vi "Main.vi"(11 "Module Admin":refnum<class "Delacor_lib_QMH_Module Admin.lvclass">) -> ()   [LabVIEW 2019, in "ContextHelp.lvlib"]
doc: "This template is based off of the Queued Message Handler design pattern and the Queued Message Handler project template that ships with LabVIEW.\n\nThe main difference is that the queue is private to this module and communication between modules is performed via Broadcast and Request events.\n\nRequest events are wrapped in public API methods and are handled in the Event Handling Loop (EHL) of this VI. Any module can register for Broadcast events sent by this module. The EHL generates messages based on user interface actions.\n\nThe Message Handling Loop (MHL) processes messages generated by the EHL, or by other messages. The messages are string values, so new messages can be added easily to the Message Cases case structure in the MHL. Each message cluster can also provide an optional value for Message Data, which is a variant that can be converted to whatever message-specific data is required.\n_____\nBased on DQMH Project Template 6.1.0.94.\n____\nPantherLAB Templates 1.0.0.5\nCopyright (c) 2022, PantherLAB"
uses:
  ContextHelp.lvlib
  <vilib>/Delacor/Delacor QMH/Libraries/Module Admin_class/Delacor_lib_QMH_Module Admin.lvclass
  Module Data--cluster.ctl
  <vilib>/Delacor/Delacor QMH/Libraries/Message Queue_class/Delacor_lib_QMH_Message Queue.lvclass/Delacor_lib_QMH_Message Queue.ctl
  Stop Argument--cluster.ctl
  <vilib>/Delacor/Delacor QMH/Libraries/Module Admin_class/Delacor_lib_QMH_Module Admin.lvclass/Delacor_lib_QMH_Module Admin.ctl
  Draw Panel Into Subpanel Argument--cluster.ctl
  Remove Panel from Subpanel Argument--cluster.ctl
  <vilib>/Delacor/Delacor QMH/Libraries/Message Queue_class/Delacor_lib_QMH_Enqueue Message (Single).vi
  <vilib>/Delacor/Delacor QMH/Libraries/Module Admin_class/Delacor_lib_QMH_Get External Launch.vi
  <vilib>/Utility/error.llb/Error Cluster From Error Code.vi
  <vilib>/ErrorRing/Error Ring.xnode
  <vilib>/Delacor/Delacor QMH/Libraries/Message Queue_class/Delacor_lib_QMH_Message Queue.lvclass
  Panther Dashboard/Panther Dashboard.lvlib
panel:
  out "Status":string
  out "error out":errorcluster
  out "DQMH Version":string
  in  "Edit Project Description":bool caption="Project Description"
  in  "Project Description":string
  in  "Edit Module Description":bool caption="Module Description"
  in  "Module Description":string
  in  "Edit VI":bool caption="Event Description"
  out "Event Connector Pane":picture
  in  "Event Description":string
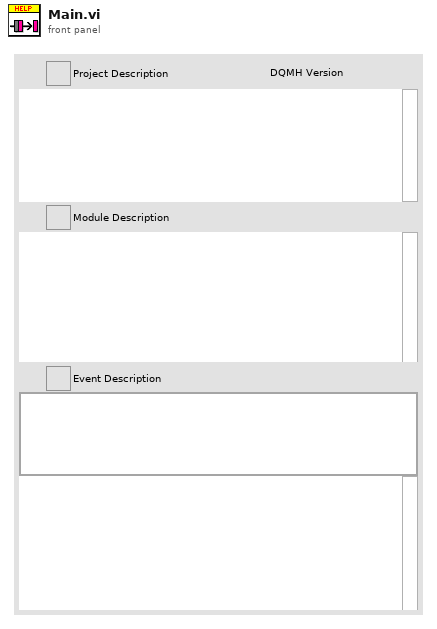
[diagram p1: front panel]
types:
  T1 = typedef "Panther Dashboard.lvlib/Broadcast Events--cluster.ctl" = cluster{"Module Did Init":refnum<user-event>, "Status Updated":refnum<user-event>, "Error Reported":refnum<user-event>, "Module Did Stop":refnum<user-event>, "Update Module Execution Status":refnum<user-event>, "References Updated":refnum<user-event>, "Projects Updated":refnum<user-event>, "Targets Updated":refnum<user-event>, "Progress updated":refnum<user-event>, "Scale Updated":refnum<user-event>, "Connector Pane Updated":refnum<user-event>, "Documentation Updated":refnum<user-event>, "Module Type Updated":refnum<user-event>, "Theme Updated":refnum<user-event>, "Project Description Updated":refnum<user-event>}
  T2 = typedef "ContextHelp.lvlib/Request Events--cluster.ctl" = cluster{"Stop Module":refnum<user-event>, "Show Panel":refnum<user-event>, "Hide Panel":refnum<user-event>, "Get Module Execution Status":refnum<user-event>, "Show Diagram":refnum<user-event>, "Draw Panel Into Subpanel":refnum<user-event>, "Remove Panel from Subpanel":refnum<user-event>, "Refresh Panther Dashboard Broadcasts":refnum<user-event>}
  T3 = typedef "ContextHelp.lvlib/Module Data--cluster.ctl" = cluster{"Status":string, "SubPanel":refnum<vi>, "Panel Status":bool}
  T4 = enum8{"Enabled", "Disabled", "Disabled and Grayed Out"}
  T5 = enum32{"invalid lock state", "Not Locked", "Locked (No Password)", "Password-protected"}
  T6 = typedef "ContextHelp.lvlib/Stop Argument--cluster.ctl" = cluster{"Origin":string, "Exit via Stop Module Req?":bool, "Wait for Module to stop?":bool}
  T7 = typedef "ContextHelp.lvlib/Draw Panel Into Subpanel Argument--cluster.ctl" = cluster{"Sub Panel":refnum<vi>}
  T8 = typedef "ContextHelp.lvlib/Remove Panel from Subpanel Argument--cluster.ctl" = cluster{"Boolean":bool}
  T9 = enum32{"Invalid", "Standard", "Closed", "Hidden", "Minimized", "Maximized"}
  T10 = typedef "Panther Dashboard.lvlib/Documentation--cluster.ctl" = cluster{"Module Description":string, "Event Description":string}
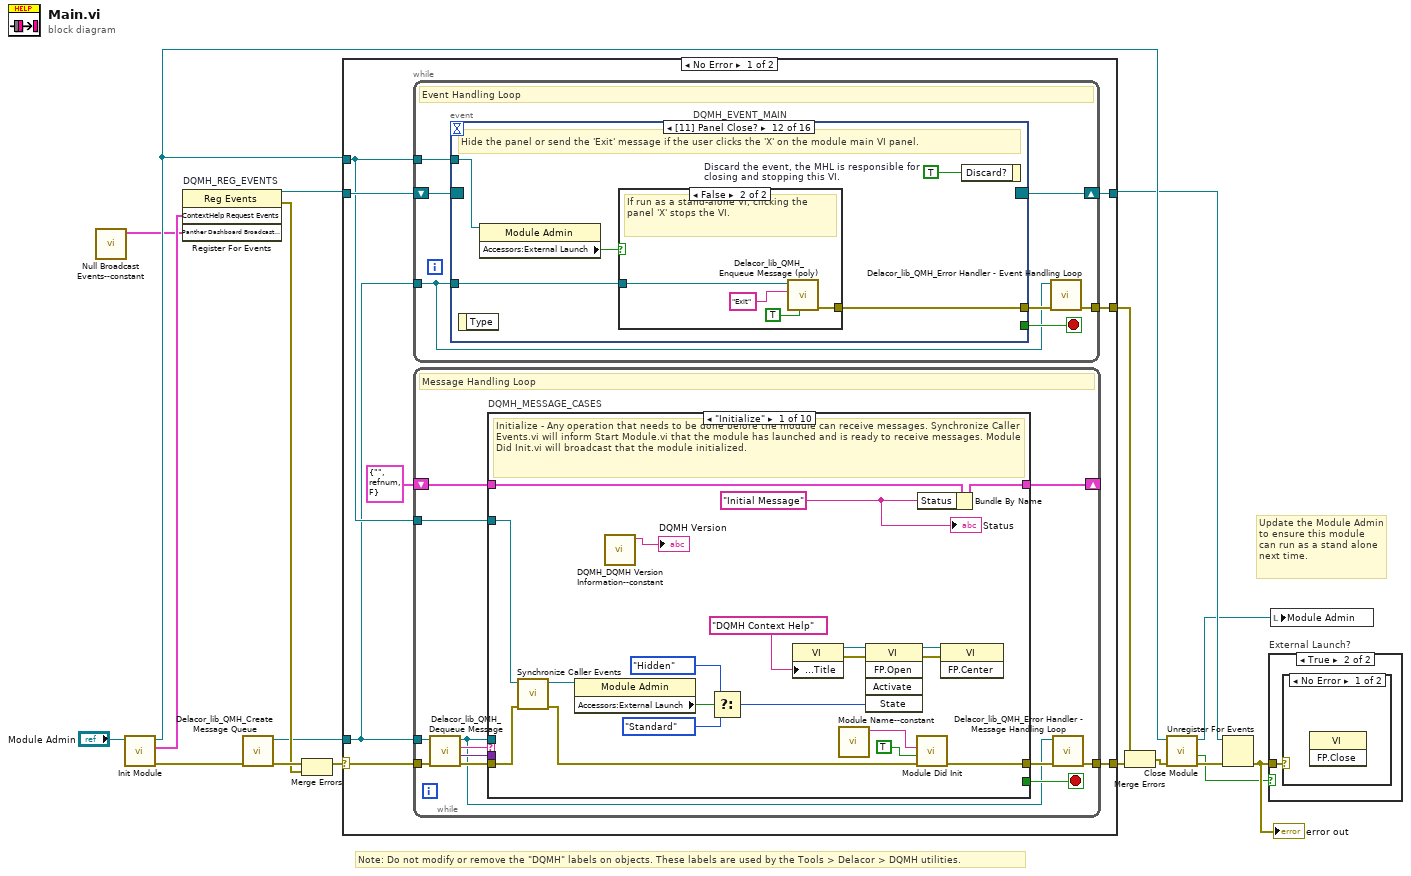
[diagram p0: block diagram]
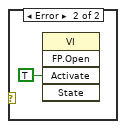
[diagram p3: hidden frame]
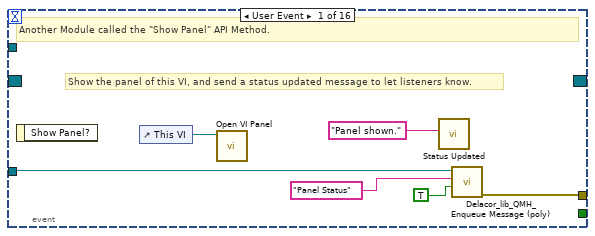
[diagram p4: hidden frame]
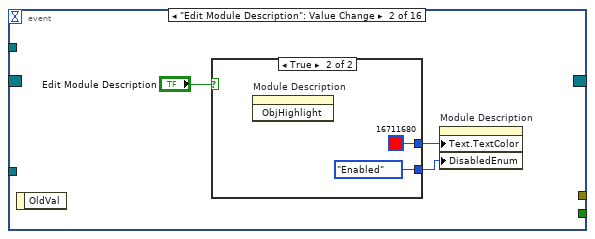
[diagram p5: hidden frame]
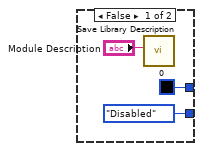
[diagram p6: hidden frame]
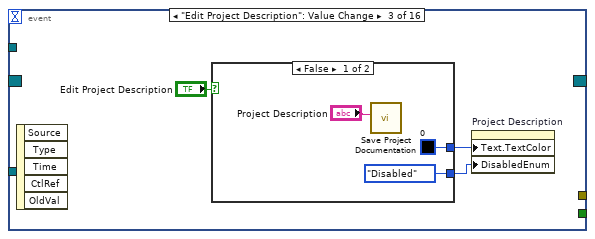
[diagram p7: hidden frame]
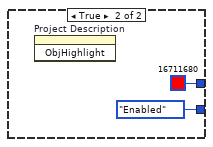
[diagram p8: hidden frame]
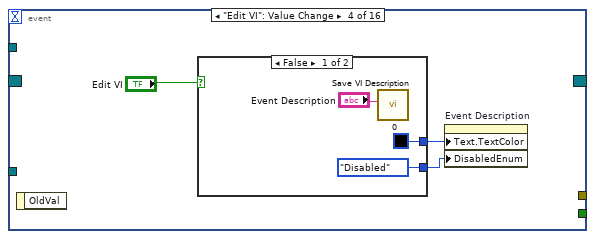
[diagram p9: hidden frame]
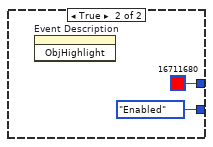
[diagram p10: hidden frame]
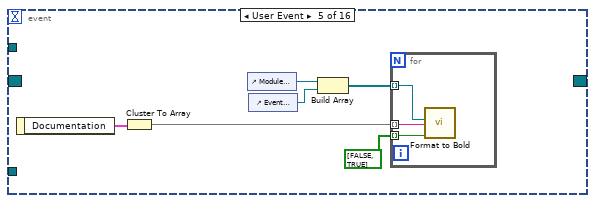
[diagram p11: hidden frame]
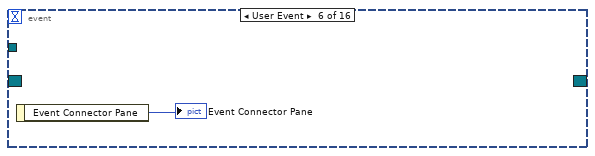
[diagram p12: hidden frame]
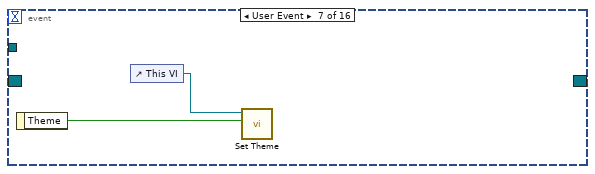
[diagram p13: hidden frame]
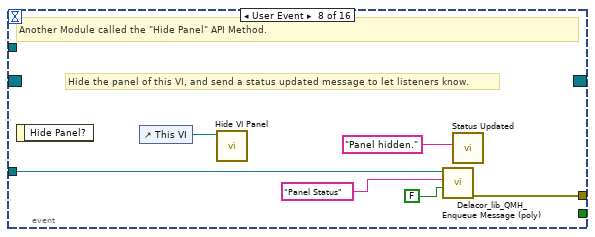
[diagram p14: hidden frame]
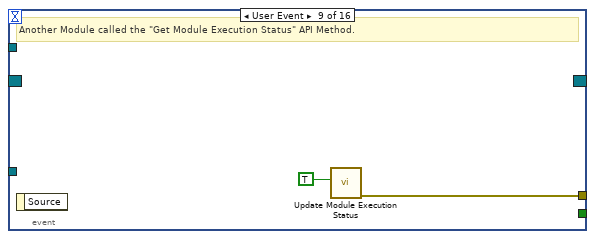
[diagram p15: hidden frame]
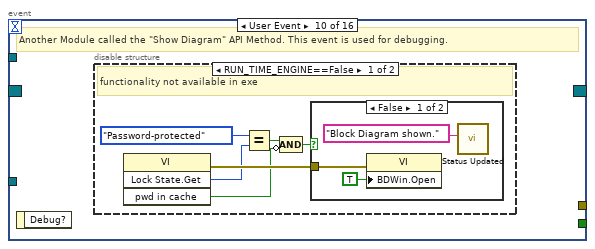
[diagram p16: hidden frame]
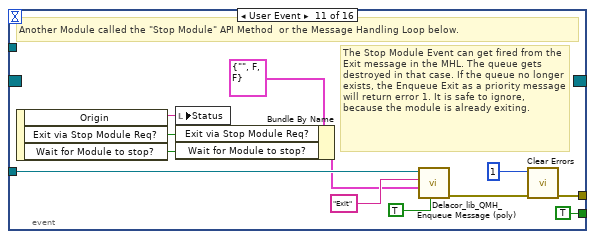
[diagram p19: hidden frame]
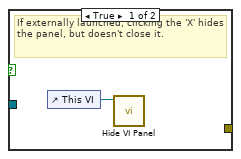
[diagram p20: hidden frame]
diagram:
  # "Note: Do not modify or remove the \"DQMH\" labels on objects. These labels are used by the Tools > Delacor > DQMH utilities."
  # "Update the Module Admin to ensure this module can run as a stand alone next time."
  n1 = call "Null Broadcast Events--constant.vi"() -> ("Panther Dashboard Broadcast Events"=w1:T1)  [unwired: 11 in]
  n2 = call "Init Module.vi"("Singleton Module Admin in"="Module Admin") -> ("error out"=w17:errorcluster, "ContextHelp Request Events"=w2:T2, "Singleton Module Admin out"=w9:refnum<class "Delacor_lib_QMH_Module Admin.lvclass">)  [unwired: 8 in]
  n3 = register-events "DQMH_REG_EVENTS"(w2, w1) -> (reference out=w7:refnum<event-registration>, error out=w10:errorcluster)  [unwired: 2 in]
  n4 = call <vilib>:"Delacor_lib_QMH_Create Message Queue.vi"("error in"=w17) -> ("error out"=w12:errorcluster, "Message Queue"=w6:refnum<class "Delacor_lib_QMH_Message Queue.lvclass">)  [unwired: 9 in]
  n5 = Merge Errors(w12, w10) -> (w11:errorcluster)
  n6 = case shown="No Error" w11 {
    selector: w11 -> [w24 w252]
    tunnel: [w26 w251] -> w18
    tunnel: [w23 w250] -> w8
    tunnel: w7 -> [w21 w250]
    tunnel: w6 -> [w19 w245]
    tunnel: [w25 _] -> w15
    tunnel: w9 -> [w20 w246]
    frame No Error {
      n7 = while {
        tunnel: w19 -> [w27]
        shift-right: [w30] -> w23
        shift-left: w21 -> [w31]
        tunnel: [w32] -> w25
        tunnel: w20 -> [w28]
        stop <- w29 stop-if-true
        # "Event Handling Loop"
        n8 = event "DQMH_EVENT_MAIN" shown="[11] Panel Close?" {
          selector: w31 -> [_ _ _ _ _ _ _ _ _ _ _ _ _ _ w129 _]
          dyn-events: [_ _ _ _ _ _ _ _ _ _ _ _ _ _ w128 _] -> w30
          timeout: _ -> [_ _ _ _ _ _ _ _ _ _ _ _ _ _ _ _]
          tunnel: [_ _ _ _ _ _ _ _ _ _ TRUE ("Discard?") _ _ _ _ _] -> w29
          tunnel: w27 -> [w36 _ _ _ _ _ _ w76 _ _ w100 w107 w119 w125 _ _]
          tunnel: [w39 _ _ _ _ _ _ w81 w83 _ w103 w109 w120 w126 _ _] -> w33
          tunnel: w28 -> [_ _ _ _ _ _ _ _ _ _ _ w106 _ _ _ _]
          event User Event {
            # "Show the panel of this VI, and send a status updated message to let listeners know."
            # "Another Module called the \"Show Panel\" API Method."
            n9 = event-data() -> ()  [unwired: 1 in, 1 out]
            n10 = control-ref of="This VI"() -> (w38:refnum<vi>)
            n11 = call "Open VI Panel.vi"("VI"=w38) -> ()  [unwired: 10 in, 1 out]
            n12 = call "Status Updated.vi"("Status"="Panel shown." ("format string")) -> ()  [unwired: 10 in, 1 out]
            n13 = call-poly <vilib>:"Delacor_lib_QMH_Enqueue Message (poly).vi"("Message Data"=TRUE, "Message"="Panel Status" ("format string"), "Message Queue in"=w36) -> ("error out"=w39:errorcluster)  [unwired: 7 in, 1 out]
          }
          event "Edit Module Description": Value Change {
            n14 = event-data() -> ()  [unwired: 1 in, 1 out]
            n15 = case shown="True" "Edit Module Description" {
              tunnel: [u32 0 u32 16711680] -> w41
              tunnel: [T4."Disabled" ("Disabled") T4."Enabled" ("Disabled")] -> w42
              frame False {
                n16 = call "Save Library Description.vi"("Library Description"="Module Description") -> ()  [unwired: 10 in, 1 out]
              }
              frame True {
                n17 = invoke on="Module Description" class="Str" method="ObjHighlight"() -> ()  [unwired: 3 in, 3 out]
              }
            }
            n18 = property on="Module Description" class="Str"("Text.TextColor"=w41, "DisabledEnum"=w42) -> ()  [unwired: 2 in, 2 out]
          }
          event "Edit Project Description": Value Change {
            n19 = event-data() -> ()  [unwired: 1 in, 5 out]
            n20 = case shown="False" "Edit Project Description" {
              tunnel: [u32 0 u32 16711680] -> w49
              tunnel: [T4."Disabled" ("Disabled") T4."Enabled" ("Disabled")] -> w50
              frame False {
                n21 = call "Save Project Documentation.vi"("Project Description"="Project Description") -> ()  [unwired: 10 in, 1 out]
              }
              frame True {
                n22 = invoke on="Project Description" class="Str" method="ObjHighlight"() -> ()  [unwired: 3 in, 3 out]
              }
            }
            n23 = property on="Project Description" class="Str"("Text.TextColor"=w49, "DisabledEnum"=w50) -> ()  [unwired: 2 in, 2 out]
          }
          event "Edit VI": Value Change {
            n24 = event-data() -> ()  [unwired: 1 in, 1 out]
            n25 = case shown="False" "Edit VI" {
              tunnel: [u32 0 u32 16711680] -> w57
              tunnel: [T4."Disabled" ("Disabled") T4."Enabled" ("Disabled")] -> w58
              frame False {
                n26 = call "Save VI Description.vi"("VI Description"="Event Description") -> ()  [unwired: 10 in, 1 out]
              }
              frame True {
                n27 = invoke on="Event Description" class="Str" method="ObjHighlight"() -> ()  [unwired: 3 in, 3 out]
              }
            }
            n28 = property on="Event Description" class="Str"("Text.TextColor"=w57, "DisabledEnum"=w58) -> ()  [unwired: 2 in, 2 out]
          }
          event User Event {
            n29 = event-data() -> ("Documentation"=w69:T10)  [unwired: 1 in]
            n30 = Cluster To Array(cluster=w69) -> (array=w67:string[])
            n31 = control-ref of="Module Description"() -> (w65:refnum<vi>)
            n32 = control-ref of="Event Description"() -> (w64:refnum<vi>)
            n33 = Build Array(w65, w64) -> (w66:refnum<vi>[])
            n34 = for {
              tunnel: bool[] [FALSE, TRUE] ("Adjust Height?") -> [w72] mode=indexing
              tunnel: w67 -> [w71] mode=indexing
              tunnel: w66 -> [w70] mode=indexing
              n35 = call "Format to Bold.vi"("Adjust Height?"=w72, "String Value"=w71, "String Ref"=w70) -> ()  [unwired: 9 in]
            }
          }
          event User Event {
            n36 = event-data() -> ("Event Connector Pane"=→"Event Connector Pane":picture)  [unwired: 1 in]
          }
          event User Event {
            n37 = event-data() -> ("Theme"=w74:bool)  [unwired: 1 in]
            n38 = control-ref of="This VI"() -> (w75:refnum<vi>)
            n39 = call "Set Theme.vi"("Dark?"=w74, "VI in"=w75) -> ()  [unwired: 10 in]
          }
          event User Event {
            # "Hide the panel of this VI, and send a status updated message to let listeners know."
            # "Another Module called the \"Hide Panel\" API Method."
            n40 = event-data() -> ()  [unwired: 1 in, 1 out]
            n41 = control-ref of="This VI"() -> (w80:refnum<vi>)
            n42 = call "Hide VI Panel.vi"("VI"=w80) -> ()  [unwired: 10 in, 1 out]
            n43 = call-poly <vilib>:"Delacor_lib_QMH_Enqueue Message (poly).vi"("Message Data"=FALSE, "Message"="Panel Status" ("format string"), "Message Queue in"=w76) -> ("error out"=w81:errorcluster)  [unwired: 7 in, 1 out]
            n44 = call "Status Updated.vi"("Status"="Panel hidden." ("format string")) -> ()  [unwired: 10 in, 1 out]
          }
          event User Event {
            # "Another Module called the \"Get Module Execution Status\" API Method."
            n45 = event-data() -> ()  [unwired: 1 in, 1 out]
            n46 = call "Update Module Execution Status.vi"("Running?"=TRUE) -> ("error out"=w83:errorcluster)  [unwired: 10 in]
          }
          event User Event {
            # "Another Module called the \"Show Diagram\" API Method. This event is used for debugging."
            n47 = event-data() -> ()  [unwired: 1 in, 1 out]
            n48 = disable-structure shown="RUN_TIME_ENGINE==False" {
              frame condition #0 (active) {
                # "functionality not available in exe"
                n49 = invoke class="VI" method="Lock State.Get"() -> (error out=w89:errorcluster, "Get Lock State"=w88:T5, "pwd in cache"=w85:bool)  [unwired: 4 in, 1 out]
                n50 = Equal?(x=T5."Password-protected", y=w88) -> (x = y?=w86:bool)
                n51 = Compound Arithmetic op=AND(w86, invert w85) -> (w84:bool)
                n52 = case shown="False" w84 {
                  tunnel: w89 -> [w92 _]
                  frame False {
                    n53 = property class="VI"(error in=w92, "BDWin.Open"=TRUE ("Block Diagram Window:Open")) -> ()  [unwired: 1 in, 2 out]
                    n54 = call "Status Updated.vi"("Status"="Block Diagram shown." ("format string")) -> ()  [unwired: 10 in, 1 out]
                  }
                  frame True {
                    # "Password-protected VI, and the password is not in the cache. Do not show the diagram."
                  }
                }
              }
              frame condition #1 {
              }
            }
          }
          event User Event {
            # "The Stop Module Event can get fired from the Exit message in the MHL. The queue gets destroyed in that case. If the queue no longer exists, the Enqueue Exit as a priority message will return error 1. It is safe to ignore, because the module is already exiting."
            # "Another Module called the \"Stop Module\" API Method  or the Message Handling Loop below."
            n55 = event-data() -> ("Origin"=w99:string, "Exit via Stop Module Req?"=w95:bool, "Wait for Module to stop?"=w94:bool)  [unwired: 1 in]
            n56 = local write "Status"(w99) -> ()
            n57 = Bundle By Name(cluster=T6 {"Origin"="", "Exit via Stop Module Req?"=FALSE, "Wait for Module to stop?"=FALSE} ("Stop Argument"), "Exit via Stop Module Req?"=w95, "Wait for Module to stop?"=w94) -> (w93:T6)
            n58 = call-poly <vilib>:"Delacor_lib_QMH_Enqueue Message (poly).vi"("Priority Message? (F)"=TRUE, "Message Data"=w93, "Message"="Exit", "Message Queue in"=w100) -> ("error out"=w104:errorcluster)  [unwired: 6 in, 1 out]
            n59 = call <vilib>:"Clear Errors.vi"("error in (no error)"=w104, "specific error code to clear (0: all)"=1) -> ("error out"=w103:errorcluster)  [unwired: 4 in, 1 out]
          }
          event Panel Close? {
            w108 = TRUE  # Discard the event, the MHL is responsible for closing and stopping this VI.
            # "Hide the panel or send the 'Exit' message if the user clicks the 'X' on the module main VI panel."
            n60 = event-data() -> ()  [unwired: 1 in, 1 out]
            n61 = property class="Module Admin"(reference=w106) -> ("Accessors:External Launch"=w105:bool)  [unwired: 1 in, 2 out]
            n62 = case shown="False" w105 {
              tunnel: w107 -> [_ w113]
              tunnel: [_ w114] -> w109
              frame True {
                # "If externally launched, clicking the 'X' hides the panel, but doesn't close it."
                n63 = control-ref of="This VI"() -> (w110:refnum<vi>)
                n64 = call "Hide VI Panel.vi"("VI"=w110) -> ()  [unwired: 10 in, 1 out]
              }
              frame False {
                # "If run as a stand-alone VI, clicking the panel 'X' stops the VI."
                n65 = call-poly <vilib>:"Delacor_lib_QMH_Enqueue Message (poly).vi"("Priority Message? (F)"=TRUE, "Message"="Exit", "Message Queue in"=w113) -> ("error out"=w114:errorcluster)  [unwired: 7 in, 1 out]
              }
            }
            n66 = event-data("Discard?"=w108) -> ()  [unwired: 1 in, 1 out]
          }
          event User Event {
            # "Another Module called the \"Draw your Panel into Subpanel\" API Method."
            n67 = event-data() -> ("Sub Panel"=w115:refnum<vi>)  [unwired: 1 in]
            n68 = Bundle(cluster=T7 {"Sub Panel"=refnum} ("Draw your Panel into Subpanel Argument"), "Sub Panel"=w115) -> (w116:T7)
            n69 = call-poly <vilib>:"Delacor_lib_QMH_Enqueue Message (poly).vi"("Message Data"=w116, "Message"="Draw Panel into Subpanel", "Message Queue in"=w119) -> ("error out"=w120:errorcluster)  [unwired: 7 in, 1 out]
          }
          event User Event {
            # "Another Module called the \"Remove Panel from Subpanel\" API Method."
            n70 = event-data() -> ("Boolean"=w121:bool)  [unwired: 1 in]
            n71 = Bundle(cluster=T8 {"Boolean"=FALSE} ("Remove Panel from Subpanel Argument"), "Boolean"=w121) -> (w122:T8)
            n72 = call-poly <vilib>:"Delacor_lib_QMH_Enqueue Message (poly).vi"("Message Data"=w122, "Message"="Remove Panel from Subpanel", "Message Queue in"=w125) -> ("error out"=w126:errorcluster)  [unwired: 7 in, 1 out]
          }
          event User Event {
            # "Another Module called the \"Refresh Panther Dashboard Broadcasts\" API Method."
            n73 = event-data() -> ()  [unwired: 1 in, 1 out]
            n74 = call "Obtain Broadcast Events for Registration.vi"() -> ("Panther Dashboard Broadcast Events"=w127:T1)  [unwired: 9 in, 2 out]
            n75 = register-events "Refresh Panther Broadcasts"(reference=w129, w127) -> (reference out=w128:refnum<event-registration>)  [unwired: 2 in, 1 out]
          }
          event User Event {
            n76 = event-data() -> ("Project Description"=w130:string)  [unwired: 1 in]
            n77 = local write "Project Description"(w130) -> ()
          }
        }
        n78 = call-dynamic "Delacor_lib_QMH_Error Handler - Event Handling Loop.vi"("error in"=w33, "Message Queue in"=w27) -> ("dup error in"=w32:errorcluster)  [unwired: 8 in, 1 out]
      }
      n79 = while {
        tunnel: w19 -> [w133]
        shift-right: [w137] -> _
        shift-left: T3 {"Status"="", "SubPanel"=refnum, "Panel Status"=FALSE} ("Data Cluster") -> [w138]
        tunnel: w24 -> [w141]
        tunnel: [w139] -> w26
        tunnel: w20 -> [w131]
        stop <- w136 stop-if-true
        # "Message Handling Loop"
        n80 = call-dynamic "Delacor_lib_QMH_Dequeue Message.vi"("error in"=w141, "Message Queue in"=w133) -> ("error out"=w140:errorcluster, "Message Data"=w134:variant, "Message"=w135:string, "Message Queue out"=w132:refnum<class "Delacor_lib_QMH_Message Queue.lvclass">)  [unwired: 6 in]
        n81 = case "DQMH_MESSAGE_CASES" shown="\"Initialize\"" w135 {
          selector: w135 -> [_ _ _ _ _ _ _ _ _ w232]
          tunnel: w132 -> [_ _ _ _ _ _ _ w201 w224 _]
          tunnel: w140 -> [w160 w164 w175 w184 w193 w196 w198 w208 w230 w234]
          tunnel: [w158 w164 w173 w183 w192 w195 w198 w204 w227 w235] -> w142
          tunnel: w138 -> [w150 w163 w172 w179 w191 w194 w197 w203 w216 w233]
          tunnel: [w149 w163 w166 w179 w188 w194 w197 w203 w216 w233] -> w137
          tunnel: [_ _ _ _ _ _ _ _ w223 _] -> w136
          tunnel: w134 -> [_ _ w171 w181 w190 _ _ w202 w222 _]
          tunnel: w131 -> [w151 _ _ _ _ _ _ w200 w217 _]
          frame "Initialize" {
            w145 = "Initial Message" ("Initial Message")
            # "Initialize - Any operation that needs to be done before the module can receive messages. Synchronize Caller Events.vi will inform Start Module.vi that the module has launched and is ready to receive messages. Module Did Init.vi will broadcast that the module initialized."
            n82 = call "Synchronize Caller Events.vi"("error in (no error)"=w160, "Singleton Module Admin in"=w151) -> ("error out"=w159:errorcluster, "Singleton Module Admin out"=w146:refnum<class "Delacor_lib_QMH_Module Admin.lvclass">)  [unwired: 8 in]
            n83 = property class="Module Admin"(reference=w146) -> ("Accessors:External Launch"=w155:bool)  [unwired: 1 in, 2 out]
            n84 = call <vilib>:"DQMH_DQMH Version Information--constant.vi"() -> ("DQMH Version"=→"DQMH Version":string)  [unwired: 11 in]
            n85 = Select(t=T9."Hidden" ("State"), s=w155, f=T9."Standard" ("State")) -> (s? t:f=w152:T9)
            n86 = property class="VI"("Front Panel.Title"="DQMH Context Help" ("Front Panel Window:Title")) -> (reference out=w157:refnum<vi>, error out=w162:errorcluster)  [unwired: 2 in]
            n87 = call "Module Name--constant.vi"() -> ("Module Name"=w147:string)  [unwired: 11 in]
            n88 = invoke class="VI" method="FP.Open"(reference=w157, error in=w162, "State"=w152) -> (reference out=w156:refnum<vi>, error out=w161:errorcluster)  [unwired: 2 in, 3 out]
            n89 = call "Module Did Init.vi"("error in (no error)"=w159, "Initialized?"=TRUE, "Origin"=w147) -> ("error out"=w158:errorcluster)  [unwired: 8 in]
            n90 = Bundle By Name(cluster=w150, "Status"=w145) -> (w149:T3)
            n91 = invoke class="VI" method="FP.Center"(reference=w156, error in=w161) -> ()  [unwired: 1 in, 3 out]
            "Status" <- w145
          }
          frame "---Module Specific---" {
            # "Separator -- The following cases handle messages specific to this Module."
          }
          frame "Draw Panel into Subpanel" {
            # "#PantherLAB_How_To\nThis module request allows to draw Main.vi into any \nsubpanel provided"
            # "Request made to the module to draw itself into a subpanel provided"
            n92 = Variant To Data(error in=w175, type=T7 {"Sub Panel"=refnum} ("Draw your Panel into Subpanel Argument"), Variant=w171) -> (data=w169:T7, error out=w174:errorcluster)
            n93 = Unbundle By Name(w169) -> ("Sub Panel"=w167:refnum<vi>)
            n94 = control-ref of="This VI"() -> (w168:refnum<vi>)
            n95 = call "Draw Panel Into Subpanel Procedure.vi"("error in"=w174, "SubPanel in"=w167, "This VI"=w168) -> ("error out"=w173:errorcluster, "SubPanel out"=w165:refnum<vi>)  [unwired: 7 in]
            n96 = Bundle By Name(cluster=w172, "SubPanel"=w165) -> (w166:T3)
          }
          frame "Remove Panel from Subpanel" {
            # "Request to the module to remove itself from the subpanel"
            n97 = Variant To Data(error in=w184, type=T8 {"Boolean"=FALSE} ("Remove Panel from Subpanel Argument"), Variant=w181) -> (error out=w183:errorcluster)  [unwired: 1 out]
            n98 = Unbundle By Name(w179) -> ("Panel Status"=w177:bool, "SubPanel"=w178:refnum<vi>)
            n99 = invoke class="SubPnl" method="Remove VI"(reference=w178) -> (error out=w182:errorcluster)  [unwired: 2 in, 2 out]
            n100 = control-ref of="This VI"() -> (w176:refnum<vi>)
            n101 = case shown="False" w177 {
              tunnel: w182 -> [_ _]
              tunnel: w176 -> [w185 w186]
              frame False {
                # "Hiden"
                n102 = call "Hide VI Panel.vi"("VI"=w185) -> ()  [unwired: 10 in, 1 out]
              }
              frame True {
                # "Visible"
                n103 = call "Open VI Panel.vi"("VI"=w186) -> ()  [unwired: 10 in, 1 out]
              }
            }
          }
          frame "Panel Status" {
            n104 = Variant To Data(error in=w193, type=TRUE, Variant=w190) -> (data=w187:bool, error out=w192:errorcluster)
            n105 = Bundle By Name(cluster=w191, "Panel Status"=w187) -> (w188:T3)
          }
          frame "---Copy This Frame---" {
            # "Duplicate this frame when creating new messages.  Change this comment in the duplicated frame to describe this message."
            n106 = Merge Errors(w196) -> (w195:errorcluster)
          }
          frame "---Exit and Error Handling---" {
            # "Separator - The following cases handle errors and exit messages."
          }
          frame "Error" {
            # "Error - Check the error message data and respond accordingly. This message is sent by the \"Error Handler\" VIs at the end of each loop in this application."
            n107 = property class="Module Admin"(reference=w200) -> ("Accessors:External Launch"=w199:bool)  [unwired: 1 in, 2 out]
            n108 = Variant To Data(error in=w208, type=errorcluster {"status"=FALSE, "code"=0, "source"=""} ("error constant"), Variant=w202) -> (data=w209:errorcluster, error out=w206:errorcluster)
            n109 = call "Error Reported.vi"("Error"=w209) -> ()  [unwired: 10 in, 1 out]
            n110 = case shown="False" w199 {
              tunnel: [w214 _] -> w205
              tunnel: w201 -> [w212 _]
              tunnel: w209 -> [w213 _]
              frame False {
                # "If the module is running standalone, then pop up an error dialog and call the \"Exit\" message."
                n111 = call <vilib>:"Simple Error Handler.vi"("error in (no error)"=w213) -> ()  [unwired: 4 in, 5 out]
                n112 = call-poly <vilib>:"Delacor_lib_QMH_Enqueue Message (poly).vi"("Priority Message? (F)"=TRUE, "Message"="Exit", "Message Queue in"=w212) -> ("error out"=w214:errorcluster)  [unwired: 7 in, 1 out]
              }
              frame True {
                # "If the module was launched externally, calling the Error Reported broadcast VI is the only action performed by the \"Error\" message. The module's caller can then process the error appropriately."
              }
            }
            n113 = Merge Errors(w206, w205) -> (w204:errorcluster)
            n114 = local write "error out"(w204) -> ()
          }
          frame "Exit" {
            w221 = 91  # 91: not all Exit messages will have an argument
            w223 = TRUE  # Stop the VI
            # "Release the message queue reference"
            # "Exit - Exit the application."
            n115 = Variant To Data(error in=w230, type=T6 {"Origin"="", "Exit via Stop Module Req?"=FALSE, "Wait for Module to stop?"=FALSE} ("Stop Argument"), Variant=w222) -> (data=w219:T6, error out=w226:errorcluster)
            n116 = call <vilib>:"Clear Errors.vi"("error in (no error)"=w226, "specific error code to clear (0: all)"=w221) -> ("error out"=w229:errorcluster)  [unwired: 4 in, 1 out]
            n117 = Unbundle By Name(w216) -> ("SubPanel"=w215:refnum<vi>)
            n118 = control-ref of="This VI"() -> (w218:refnum<vi>)
            n119 = invoke class="SubPnl" method="Remove VI"(reference=w215) -> ()  [unwired: 2 in, 3 out]
            n120 = call-dynamic "Delacor_lib_QMH_Release Message Queue.vi"("error in"=w229, "Message Queue"=w224) -> ("error out"=w228:errorcluster)  [unwired: 9 in]
            n121 = call "Handle Exit.vi"("Stop Argument"=w219, "Admin in"=w217, "VI reference"=w218) -> ("error out"=w225:errorcluster)  [unwired: 7 in, 1 out]
            n122 = Merge Errors(w228, w225) -> (w227:errorcluster)
          }
          frame Default {
            # "'Default' case only runs if there is a message that isn't defined in any of the other cases.  Output a programming error."
            n123 = call "Module Name--constant.vi"() -> ("Module Name"=w231:string)  [unwired: 11 in]
            n124 = xnode "Error Ring"("parameter 0"=w232, "parameter 1"=w231) -> ("error out"=w236:errorcluster)
            n125 = Merge Errors(w234, w236) -> (w235:errorcluster)
          }
        }
        n126 = call-dynamic "Delacor_lib_QMH_Error Handler - Message Handling Loop.vi"("error in"=w142, "Message Queue in"=w132) -> ("dup error in"=w139:errorcluster)  [unwired: 8 in, 1 out]
      }
    }
    frame Error {
      # "Synchronize Caller Events.vi will inform Start Module.vi that the module has launched and will let the code calling Start Module.vi register for broadcasts and would permit the caller receive the broadcast that an error occurred at launch time."
      n127 = call-dynamic "Delacor_lib_QMH_Release Message Queue.vi"("error in"=w252, "Message Queue"=w245) -> ("error out"=w251:errorcluster)  [unwired: 9 in]
      n128 = call "Synchronize Caller Events.vi"("Singleton Module Admin in"=w246) -> ("error out"=w253:errorcluster)  [unwired: 9 in, 1 out]
      n129 = call "Module Name--constant.vi"() -> ("Module Name"=w249:string)  [unwired: 11 in]
      n130 = Format Into String(format string="An error occurred during initialization. %s is no longer running.", w249) -> (resulting string=w247:string)  [unwired: 2 in, 1 out]
      n131 = Merge Errors(w251, w253) -> (w254:errorcluster)
      n132 = call "Error Reported.vi"("Additional Information"=w247, "Error"=w254) -> ()  [unwired: 9 in, 1 out]
    }
  }
  n133 = Merge Errors(w15, w18) -> (w14:errorcluster)
  n134 = call "Close Module.vi"("error in (no error)"=w14, "Module Admin in"=w9) -> ("error out"=w16:errorcluster, "External Launch"=w3:bool, "Module Admin out"=w4:refnum<class "Delacor_lib_QMH_Module Admin.lvclass">)  [unwired: 7 in]
  n135 = Unregister For Events(event registration refnum=w8, error in=w16) -> (error out=w13:errorcluster)
  "error out" <- w13
  n136 = case "External Launch?" shown="True" w3 {
    tunnel: w13 -> [_ w255]
    frame False {
    }
    frame True {
      n137 = case shown="No Error" w255 {
        frame No Error {
          n138 = invoke class="VI" method="FP.Close"() -> ()  [unwired: 3 in, 3 out]
        }
        frame Error {
          n139 = invoke class="VI" method="FP.Open"("Activate"=TRUE ("Activate?")) -> ()  [unwired: 4 in, 5 out]
        }
      }
    }
  }
  n140 = local write "Module Admin"(w4) -> ()
